vi "Scan Setup.vi"(8 "error in (no error)":errorcluster, 11 "Pulse Gen Scan in":refnum<class "Pulse Gen Scan.lvclass">) -> (0 "error out":errorcluster, 3 "Pulse Gen Scan out":refnum<class "Pulse Gen Scan.lvclass">)   [LabVIEW 2012, in "Pulse Gen Scan.lvclass"]
uses:
  Pulse Gen Scan.lvclass
  Scanner/Scanner.lvclass
  Pulse Gen Scan.lvclass/Pulse Gen Scan.ctl
  Global/GPIB Numbers.vi
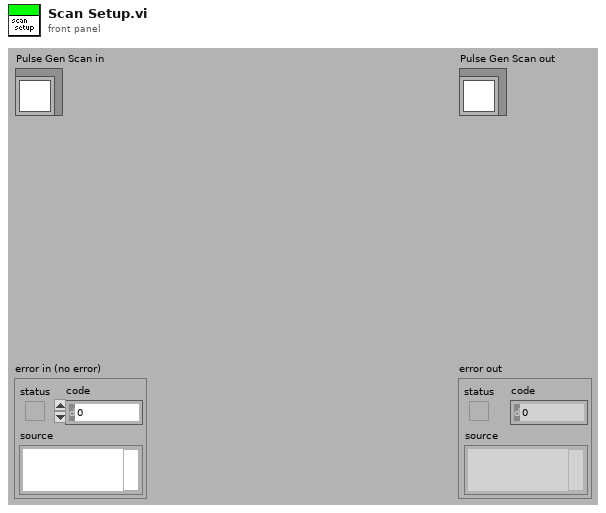
[diagram p1: front panel]
types:
  T1 = typedef "GPIB Type Def.ctl" = cluster{"Name":string, "bus":dbl, "GPIB":dbl, "GPIB as string":string, "byte":i32, "VISA Resource Name":refnum<visa-resource-name>}
  T2 = enum16{"Internal Oscillator", "Internal PLL", "Clock Input"}
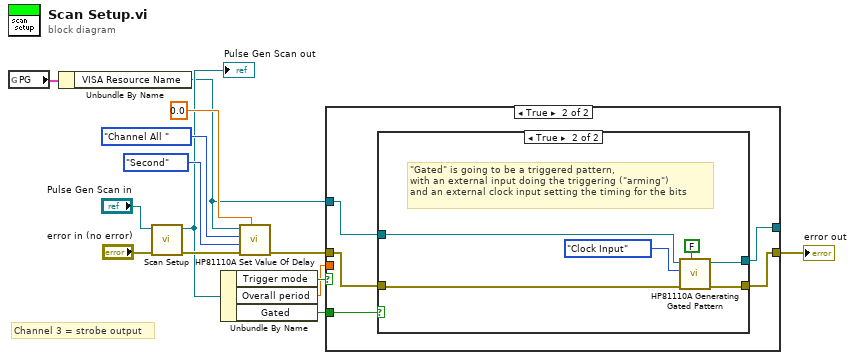
[diagram p0: block diagram]
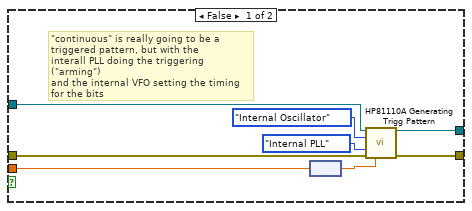
[diagram p2: hidden frame]
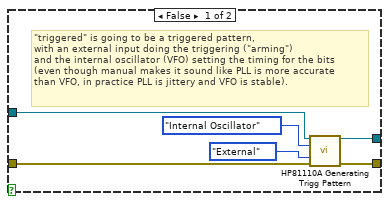
[diagram p3: hidden frame]
diagram:
  # "Channel 3 = strobe output"
  n1 = global read "GPIB Numbers.vi" "PG"() -> (w12:T1)
  n2 = Unbundle By Name(w12) -> ("VISA Resource Name"=w4:refnum<visa-resource-name>)
  n3 = call-parent "Scan Setup.vi"("error in (no error)"="error in (no error)", "Scanner in"="Pulse Gen Scan in") -> ("error out"=w8:errorcluster, "Scanner out"=w7:refnum<class "Pulse Gen Scan.lvclass">)  [unwired: 8 out]
  "Pulse Gen Scan out" <- w7
  n4 = Unbundle By Name(w7) -> ("Trigger mode"=w6:bool, "Overall period"=w5:dbl[unit], "Gated"=w2:bool)
  n5 = call "HP81110A Set Value Of Delay.vi"("Delay Value (0.0)"=0.0, "error in (no error)"=w8, "Delay Unit (0:Second)"=enum16{"Second", "Percent", "Degree", "Radians"}."Second", "Channel (1:Channel 1)"=enum16{"Channel All ", "Channel 1", "Channel 2"}."Channel All ", "VISA session"=w4) -> ("error out"=w3:errorcluster)  [unwired: 6 out]
  n6 = case shown="True" w6 {
    tunnel: w3 -> [w19 w27]
    tunnel: [w18 w23] -> w1
    tunnel: w4 -> [w20 w26]
    tunnel: w5 -> [w17 _]
    tunnel: [w15 w24] -> _
    tunnel: w2 -> [_ w25]
    frame False {
      # "\"continuous\" is really going to be a \ntriggered pattern, but with the \ninterall PLL doing the triggering (\"arming\")\nand the internal VFO setting the timing \nfor the bits"
      n7 = node(w17) -> (w16:dbl)
      n8 = call "HP81110A Generating Trigg Pattern.vi"("VISA session"=w20, "Period Source (0:Internal Oscillator)"=T2."Internal Oscillator", "Trigger Source (0:Internal PLL)"=enum16{"Internal PLL", "External", "Manual"}."Internal PLL", "error in (no error)"=w19, "PLL Value (10.0E-6)"=w16) -> ("dup VISA session"=w15:refnum<visa-resource-name>, "error out"=w18:errorcluster)  [unwired: 3 in, 6 out]
    }
    frame True {
      n9 = case shown="True" w25 {
        tunnel: w26 -> [w32 w36]
        tunnel: w27 -> [w31 w34]
        tunnel: [w30 w38] -> w23
        tunnel: [w28 w37] -> w24
        frame False {
          # "\"triggered\" is going to be a triggered pattern, \nwith an external input doing the triggering (\"arming\")\nand the internal oscillator (VFO) setting the timing for the bits \n(even though manual makes it sound like PLL is more accurate \nthan VFO, in practice PLL is jittery and VFO is stable)."
          n10 = call "HP81110A Generating Trigg Pattern.vi"("VISA session"=w32, "Period Source (0:Internal Oscillator)"=T2."Internal Oscillator", "Trigger Source (0:Internal PLL)"=enum16{"Internal PLL", "External", "Manual"}."External", "error in (no error)"=w31) -> ("dup VISA session"=w28:refnum<visa-resource-name>, "error out"=w30:errorcluster)  [unwired: 4 in, 6 out]
        }
        frame True {
          # "\"Gated\" is going to be a triggered pattern, \nwith an external input doing the triggering (\"arming\")\nand an external clock input setting the timing for the bits"
          n11 = call "HP81110A Generating Gated Pattern.vi"("Gate Source (T:Manual)"=FALSE, "error in (no error)"=w34, "Period Source (0:Internal Oscillator)"=T2."Clock Input", "VISA session"=w36) -> ("error out"=w38:errorcluster, "dup VISA session"=w37:refnum<visa-resource-name>)  [unwired: 6 in]
        }
      }
    }
  }
  "error out" <- w1
